vi "DAQ助手.vi"() -> ()   [LabVIEW 2010]
uses:
  <vilib>/measure/maspectr.llb/FFT Spectrum (Mag-Phase) for 1 Chan.vi
  <vilib>/measure/NI_MAPro.lvlib
panel:
  in  "取樣頻率(Hz)":dbl=10000.0
  out "Waveform Graph 2":waveform(dbl)(graph)
  out "Waveform Graph":cluster{"f0":dbl, "df":dbl, "magnitude":dbl[]}(graph)
  in  "stop (F)":bool
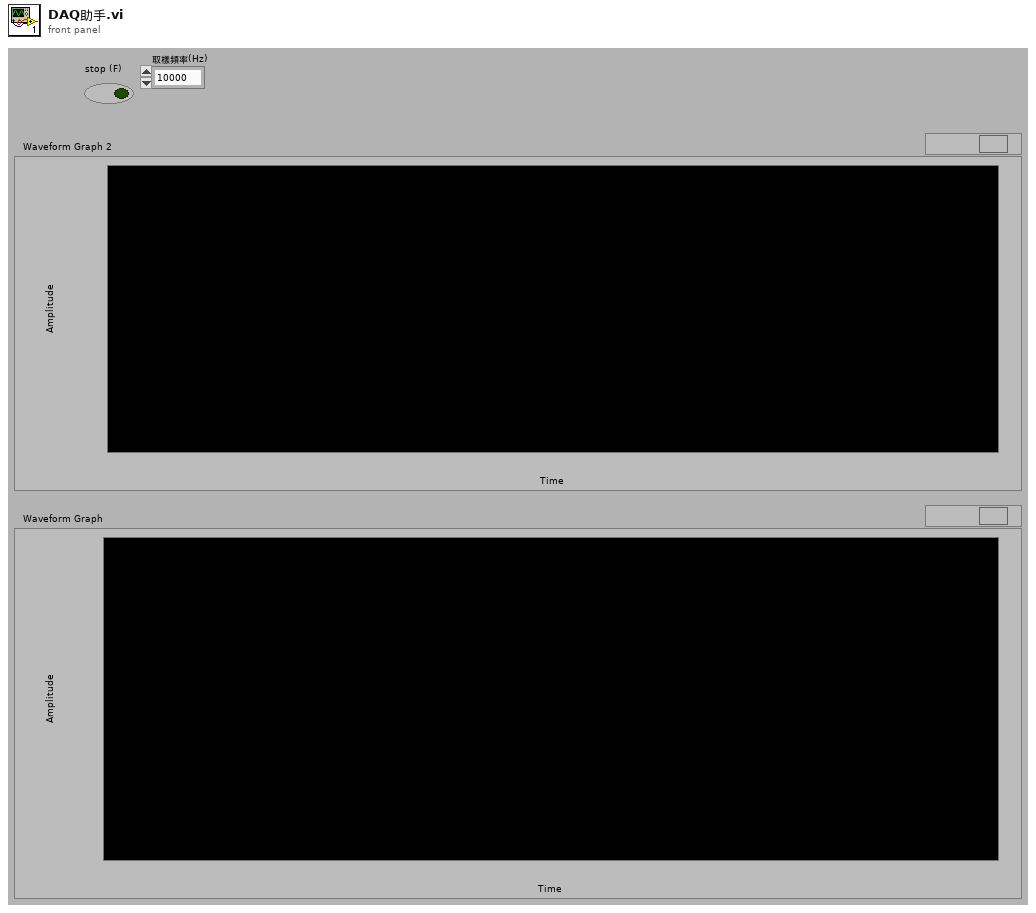
[diagram p1: front panel]
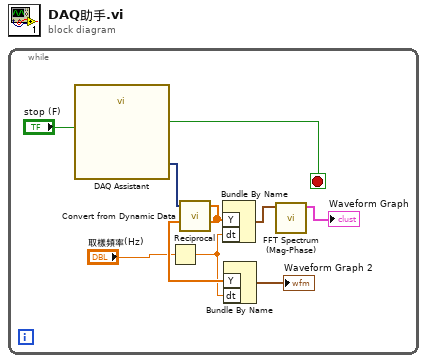
[diagram p0: block diagram]
diagram:
  n1 = while {
    stop <- w8 stop-if-true
    n2 = call "DAQ Assistant"("stop (F)"="stop (F)") -> ("data"=w7:dynamicdata, "stopped"=w8:bool)  [unwired: 15 in, 2 out]
    n3 = Reciprocal(x="取樣頻率(Hz)") -> (1/x=w1:dbl)
    n4 = call "Convert from Dynamic Data"("Dynamic Data Type"=w7) -> ("Array"=w4:dbl[])  [unwired: 3 in]
    n5 = Bundle By Name("Y"=w4, "dt"=w1) -> (w5:waveform(dbl))  [unwired: 1 in]
    n6 = Bundle By Name("Y"=w4, "dt"=w1) -> (→"Waveform Graph 2":waveform(dbl))  [unwired: 1 in]
    n7 = call-poly <vilib>:"FFT Spectrum (Mag-Phase).vi"("time signal"=w5) -> ("magnitude"=→"Waveform Graph":cluster{"f0":dbl, "df":dbl, "magnitude":dbl[]})  [unwired: 6 in, 4 out]
  }
